vi "Path.vi"(9 "error in (no error)":errorcluster, 10 "selected path":path) -> (0 "appended path":path, 1 "Exist?":bool, 2 "Boolean":bool, 3 "error out":errorcluster)   [LabVIEW 2018, in "Test_Libraries.lvlib"]
uses:
  Proyecto/Test_Libraries.lvlib
  <vilib>/Utility/file.llb/Write Delimited Spreadsheet (string).vi
panel:
  out "Name":string
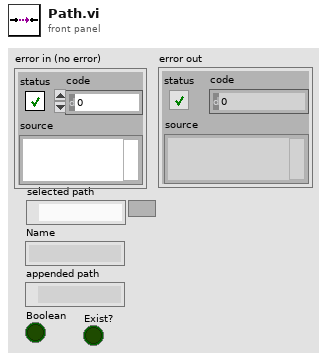
[diagram p1: front panel]
types:
  T1 = enum16{"open", "replace", "create", "open or create", "replace or create", "replace or create with confirmation"}
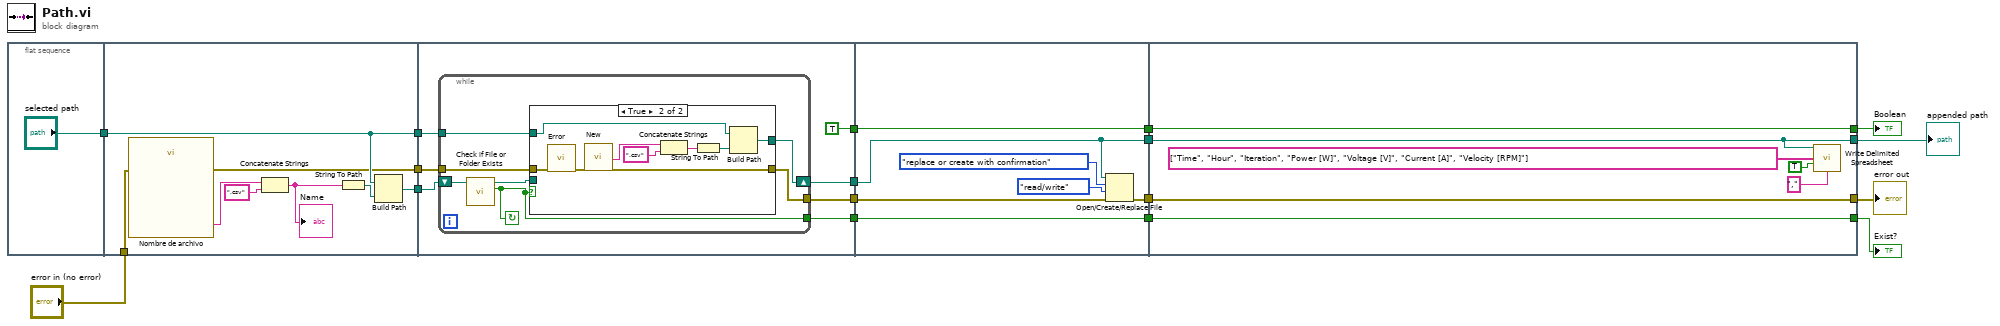
[diagram p0: block diagram]
diagram:
  n1 = flat-sequence {
    tunnel: ["selected path"] -> w17
    tunnel: w17 -> [w21]
    tunnel: [w22] -> w16
    tunnel: [w21] -> w15
    tunnel: [w20] -> w8
    tunnel: "error in (no error)" -> [w19]
    tunnel: w16 -> [w33]
    tunnel: w15 -> [w32]
    tunnel: [w31] -> w11
    tunnel: [TRUE] -> w10
    tunnel: [w29] -> w9
    tunnel: w8 -> [w28]
    tunnel: [w27] -> w7
    tunnel: w11 -> [w56]
    tunnel: w10 -> [w58]
    tunnel: w9 -> [w57]
    tunnel: w7 -> [w52]
    tunnel: [w56] -> w4
    tunnel: [w58] -> w3
    tunnel: [w57] -> w2
    tunnel: [w53] -> w1
    tunnel: [w61] -> w6
    tunnel: [w64] -> w12
    tunnel: [w65] -> w13
    tunnel: [w63] -> w14
    tunnel: w4 -> [w63]
    tunnel: w3 -> [w65]
    tunnel: w2 -> [w64]
    tunnel: w1 -> [w61]
    frame #0 {
    }
    frame #1 {
      n2 = call "Nombre de archivo"("error in (no error)"=w19) -> ("Nombre"=w26:string, "error out"=w20:errorcluster)  [unwired: 16 in, 1 out]
      n3 = Concatenate Strings(w26, ".csv" ("string")) -> (w23:string)
      "Name" <- w23
      n4 = String To Path(string=w23) -> (path=w24:path)
      n5 = Build Path(base path=w21, name or relative path=w24) -> (appended path=w22:path)
    }
    frame #2 {
      n6 = while {
        shift-right: [w38] -> w31
        shift-left: w33 -> [w40]
        tunnel: w32 -> [w39]
        tunnel: [w36] -> w29
        tunnel: w28 -> [w35]
        tunnel: [w34] -> w27
        stop <- w36 continue-if-true
        n7 = call <vilib>:"Check if File or Folder Exists.vi"("path"=w40) -> ("file or folder exists?"=w36:bool, "dup path"=w37:path)  [unwired: 8 in, 1 out]
        n8 = case shown="True" w36 {
          tunnel: w39 -> [_ w47]
          tunnel: [w42 w46] -> w38
          tunnel: w37 -> [w42 _]
          tunnel: w35 -> [w41 w44]
          tunnel: [w41 w43] -> w34
          frame False {
          }
          frame True {
            n9 = call "Error"("error in (no error)"=w44) -> ("error out"=w50:errorcluster)  [unwired: 9 in, 1 out]
            n10 = call "New"("error in (no error)"=w50) -> ("Nombre"=w45:string, "error out"=w43:errorcluster)  [unwired: 16 in, 1 out]
            n11 = Concatenate Strings(w45, ".csv" ("string")) -> (w51:string)
            n12 = String To Path(string=w51) -> (path=w48:path)
            n13 = Build Path(base path=w47, name or relative path=w48) -> (appended path=w46:path)
          }
        }
      }
    }
    frame #3 {
      n14 = Open/Create/Replace File(file path (use dialog)=w56, error in=w52, operation (0:open)=T1."replace or create with confirmation", access (0:read/write)=enum16{"read/write", "read-only", "write-only"}."read/write") -> (error out=w53:errorcluster)  [unwired: 2 in, 2 out]
    }
    frame #4 {
      n15 = call-poly <vilib>:"Write Delimited Spreadsheet.vi"("file path (dialog if empty)"=w63, "1D data"=string[] ["Time", "Hour", "Iteration", "Power [W]", "Voltage [V]", "Current [A]", "Velocity [RPM]"] ("row headers"), "append to file? (new file:F)"=TRUE, "delimiter (\\t)"="," ("delimiter (\\t)")) -> ()  [unwired: 10 in, 2 out]
    }
  }
  "appended path" <- w14
  "Boolean" <- w13
  "Exist?" <- w12
  "error out" <- w6
